vi "Configure Power Line.vi"(8 "error in (no error)":errorcluster, 10 "Frequency (0: 50 Hz)":u16(ring) items=["50 Hz", "60 Hz"], 11 "VISA resource name":refnum<visa-resource-name>) -> (0 "error out":errorcluster, 3 "VISA resource name out":refnum<visa-resource-name>)   [LabVIEW 2022 SP3, in "Agilent U2722.lvlib"]
doc: "Configures the characteristics of power line."
uses:
  Agilent U2722.lvlib
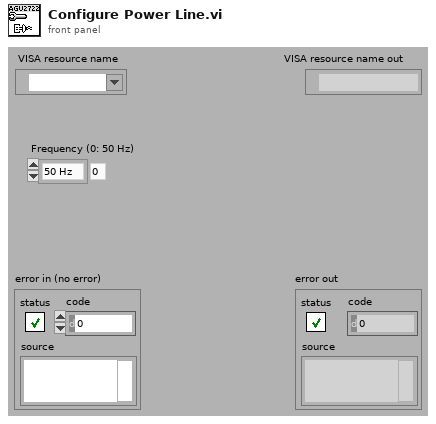
[diagram p1: front panel]
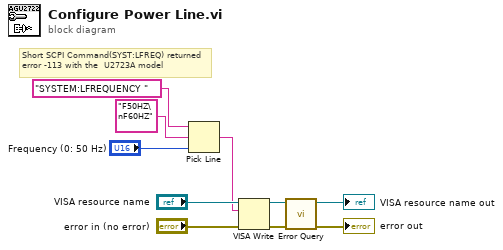
[diagram p0: block diagram]
diagram:
  # "Short SCPI Command(SYST:LFREQ) returned error -113 with the  U2723A model"
  n1 = Pick Line(string ("")="SYSTEM:LFREQUENCY ", multi-line string="F50HZ\nF60HZ", line index="Frequency (0: 50 Hz)") -> (output string=w2:string)
  n2 = VISA Write(VISA resource name="VISA resource name", write buffer=w2, error in (no error)="error in (no error)") -> (VISA resource name out=w6:refnum<visa-resource-name>, error out=w5:errorcluster)  [unwired: 1 out]
  n3 = call "Error Query.vi"("error in (no error)"=w5, "VISA resource name"=w6) -> ("error out"=→"error out":errorcluster, "VISA resource name out"=→"VISA resource name out":refnum<visa-resource-name>)  [unwired: 6 in, 2 out]
